vi "StandardSettings.vi"(3 "StandardSettings":T1={"threshold"={"max"=100, "min"=20}, "RGB or false color"=TRUE, "16bit"=TRUE, "log/lin axis"=1, "spotsize button"=TRUE, "Pixelsize"=10, "autoscale x"=TRUE, "autoscale y"=TRUE, "correlation"=TRUE, "ADC-Resolution"=128, "F2-lifetime"={"display tau"=FALSE, "display F2"=FALSE, "Palette Number lifetime"=enum."Temperature", "Palette Number F2"=enum."Rainbow", "max tau-Value"=10.0, "min tau-Value"=0.0, "max F2-Value"=1.0, "min F2-Value"=0.0}, "TAC-Window 1"=60, "TAC-Window 2"=0, "false color palette"={"1"=0, "2"=0, "3"=0, "4"=0, "5"=0, "6"=0, "7"=0, "8"=0, "8 2"=0, "8 3"=0, "8 4"=0, "8 5"=0}, "rebinning"=32.0} {"false color palette"."8 5" format="%.0x"; "false color palette"."8 4" format="%.0x"; "false color palette"."8 3" format="%.0x"; "false color palette"."8 2" format="%.0x"; "false color palette"."8" format="%.0x"; "false color palette"."7" format="%.0x"; "false color palette"."6" format="%.0x"; "false color palette"."5" format="%.0x"; "false color palette"."4" format="%.0x"; "false color palette"."3" format="%.0x"; "false color palette"."2" format="%.0x"; "false color palette"."1" format="%.0x"; "log/lin axis" items=["linear y-axis", "log y-axis"]; "F2-lifetime"."min tau-Value" format="%.2f"; "F2-lifetime"."max tau-Value" format="%.2f"; "F2-lifetime"."max F2-Value" format="%.2f"; "F2-lifetime"."min F2-Value" format="%.2f"}, 5 "Enum":enum16{"Load", "get", "Save", "set"}(ring)) -> (0 "StandardSettings":T1={"threshold"={"max"=0, "min"=0}, "RGB or false color"=TRUE, "16bit"=TRUE, "log/lin axis"=0, "spotsize button"=TRUE, "Pixelsize"=10, "autoscale x"=TRUE, "autoscale y"=TRUE, "correlation"=TRUE, "ADC-Resolution"=128, "F2-lifetime"={"display tau"=FALSE, "display F2"=FALSE, "Palette Number lifetime"=enum."Temperature", "Palette Number F2"=enum."Rainbow", "max tau-Value"=10.0, "min tau-Value"=0.0, "max F2-Value"=1.0, "min F2-Value"=0.0}, "TAC-Window 1"=60, "TAC-Window 2"=0, "false color palette"={"1"=0, "2"=0, "3"=0, "4"=0, "5"=0, "6"=0, "7"=0, "8"=0, "8 2"=0, "8 3"=0, "8 4"=0, "8 5"=0}, "rebinning"=0.0} {"false color palette"."8 5" format="%.0x"; "false color palette"."8 4" format="%.0x"; "false color palette"."8 3" format="%.0x"; "false color palette"."8 2" format="%.0x"; "false color palette"."8" format="%.0x"; "false color palette"."7" format="%.0x"; "false color palette"."6" format="%.0x"; "false color palette"."5" format="%.0x"; "false color palette"."4" format="%.0x"; "false color palette"."3" format="%.0x"; "false color palette"."2" format="%.0x"; "false color palette"."1" format="%.0x"; "log/lin axis" items=["linear y-axis", "log y-axis"]; "F2-lifetime"."min tau-Value" format="%.2f"; "F2-lifetime"."max tau-Value" format="%.2f"; "F2-lifetime"."max F2-Value" format="%.2f"; "F2-lifetime"."min F2-Value" format="%.2f"})   [LabVIEW 2009]
uses:
  Settings.ctl
  <vilib>/Utility/xml.llb/Read From XML File(string).vi
  <vilib>/Utility/xml.llb/Write to XML File(string).vi
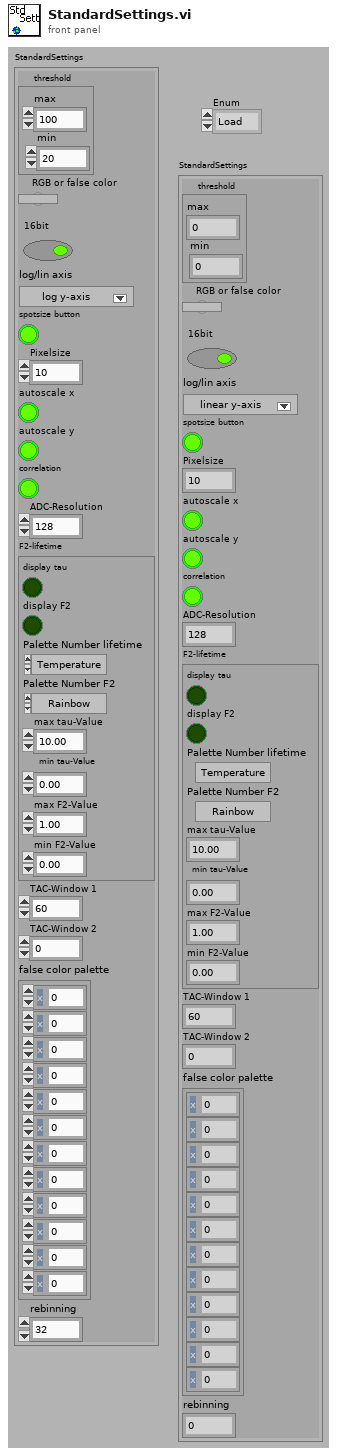
[diagram p1: front panel]
types:
  T1 = typedef "Settings.ctl" = cluster{"threshold":cluster{"max":u32, "min":u32}, "RGB or false color":bool, "16bit":bool, "log/lin axis":u16, "spotsize button":bool, "Pixelsize":u16, "autoscale x":bool, "autoscale y":bool, "correlation":bool, "ADC-Resolution":i32, "F2-lifetime":cluster{"display tau":bool, "display F2":bool, "Palette Number lifetime":enum32{"Gray", "Binary", "Gradient", "Rainbow", "Temperature"}, "Palette Number F2":enum32{"Gray", "Binary", "Gradient", "Rainbow", "Temperature"}, "max tau-Value":dbl, "min tau-Value":dbl, "max F2-Value":dbl, "min F2-Value":dbl}, "TAC-Window 1":u16, "TAC-Window 2":u16, "false color palette":cluster{"1":u32, "2":u32, "3":u32, "4":u32, "5":u32, "6":u32, "7":u32, "8":u32, "8 2":u32, "8 3":u32, "8 4":u32, "8 5":u32}, "rebinning":dbl}
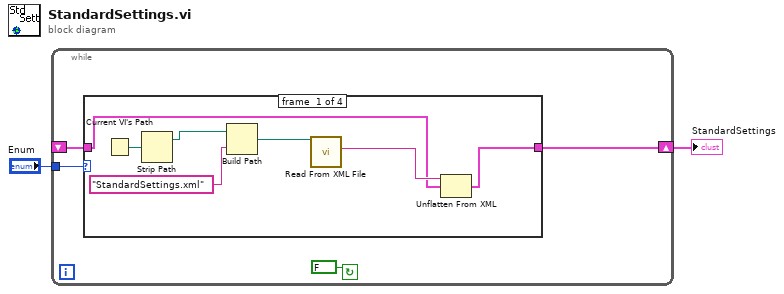
[diagram p0: block diagram]
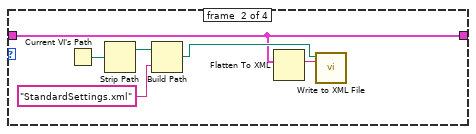
[diagram p2: hidden frame]
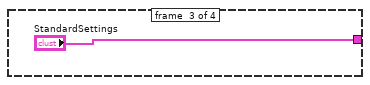
[diagram p3: hidden frame]
diagram:
  n1 = while {
    shift-right: [w3] -> w1
    shift-left: _ -> [w5]
    tunnel: "Enum" -> [w6]
    stop <- FALSE continue-if-true
    n2 = case shown="\"Save\"" w6 {
      tunnel: w5 -> [w9 w14 _ w21]
      tunnel: [w8 w14 "StandardSettings" w21] -> w3
      frame #0 {
        n3 = Current VI's Path() -> (path=w13:path)
        n4 = Strip Path(path=w13) -> (stripped path=w7:path)  [unwired: 1 out]
        n5 = Build Path(base path=w7, name or relative path="StandardSettings.xml") -> (appended path=w11:path)
        n6 = call-poly <vilib>:"Read From XML File.vi"("XML File Path"=w11) -> ("XML Elements"=w10:string)  [unwired: 8 in, 2 out]
        n7 = Unflatten From XML(xml string=w10, type=w9) -> (value=w8:T1)  [unwired: 1 in, 1 out]
      }
      frame #1 {
        n8 = Current VI's Path() -> (path=w19:path)
        n9 = Strip Path(path=w19) -> (stripped path=w17:path)  [unwired: 1 out]
        n10 = Build Path(base path=w17, name or relative path="StandardSettings.xml") -> (appended path=w15:path)
        n11 = Flatten To XML(anything=w14) -> (xml string=w16:string)
        n12 = call-poly <vilib>:"Write to XML File.vi"("XML Input"=w16, "XML File Path"=w15) -> ()  [unwired: 7 in, 3 out]
      }
      frame #2 {
      }
      frame #3 {
      }
    }
  }
  "StandardSettings" <- w1
